vi "Do.vi"(8 "error in (no error)":errorcluster, 10 "DMM":refnum<class "DMM.lvclass">, 11 "Close DMM in":refnum<class "Close DMM.lvclass">) -> (0 "error out":errorcluster, 2 "DMM":refnum<class "DMM.lvclass">, 3 "Close DMM out":refnum<class "Close DMM.lvclass">)   [LabVIEW 2020, in "Close DMM.lvclass"]
uses:
  Close DMM.lvclass
  DMM/DMM.lvclass
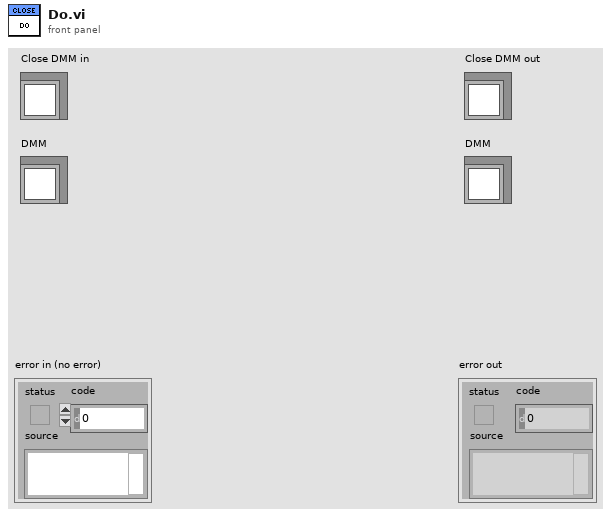
[diagram p1: front panel]
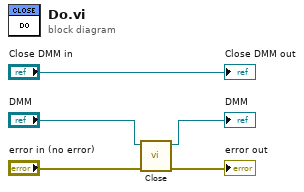
[diagram p0: block diagram]
diagram:
  n1 = call-dynamic "Close.vi"("error in (no error)"="error in (no error)", "DMM in"="DMM") -> ("error out"=→"error out":errorcluster, "DMM out"=→"DMM":refnum<class "DMM.lvclass">)  [unwired: 8 in]
  "Close DMM out" <- "Close DMM in"
